vi "Initialize Motion.vi"(7 "Motion Control":T8={"SAS Geometry"=enum."Circular", "Angular Step"=1.0, "Vertical Step"=0.0, "Vertical Min"=0.0, "Vertical Max"=0.0, "Angular Start"=1.0, "Angular Stop"=20.0}, 8 "Error In":errorcluster, 11 "AirSAS Controls":T1={"Receive Duration"=0.0, "I/O"={"DAQmx Device"="Dev1", "AO Range"=0.0, "AI Range"=0.0, "DAQ Group Delay"=0.0, "Fs"=0.0}, "Hardware"={"Centerpos"=[], "TXpos"=[], "RX1pos"=[], "RX2pos"=[], "Angle"=0.0, "Height"=0.0}, "Waveform"={"LFM Parameters"={"Duration"=1.0, "Fstart (Hz)"=1000.0, "Fstop (Hz)"=10000.0, "Out. Amplitude (Vpk)"=1.0, "Window %"=10.0}, "Transmit Waveform"={"t0"=timestamp(0 s since 1904-01-01), "dt"=1.0, "Y"=[]}}, "LINX Resource"={"IO"=enum."Remote", "Interface"=enum."Serial", "LINX Device Config"={"Interface"=enum."Serial", "COM Port"="COM13", "TCP Configuration"={"IP Address"="", "Port"=0}, "Device Family"=1, "Device ID"=1, "Device Name"="myRIO-1900", "TCP Ref"=refnum, "Channels"={"DI"=[0, 1, 2, 3, 4, 5, 6, 7, 8, 9, 10, 11, 12, 13, 14, 15, 16, 17, 18, 19, 20, 21, 22, 23, 24, 25, 26, 27, 28, 29, 30, 31, 32, 33, 34, 35, 36, 37, 38, 39, 40, 41, 42, 43, 44, 45, 46], "DO"=[0, 1, 2, 3, 4, 5, 6, 7, 8, 9, 10, 11, 12, 13, 14, 15, 16, 17, 18, 19, 20, 21, 22, 23, 24, 25, 26, 27, 28, 29, 30, 31, 32, 33, 34, 35, 36, 37, 38, 39, 40, 41, 42, 43, 44, 45, 46], "AI"=[0, 1, 2, 3, 4, 5, 6, 7, 8, 9, 10, 11], "AO"=[], "PWM"=[3, 5, 6, 9, 10], "QE"=[], "UART"=[0, 1], "I2C 2"=[0], "SPI"=[0], "CAN"=[], "Servo"=[], "AI Ref (V)"=0.0, "AI Resolution (Bits)"=0, "AO Ref (V)"=0.0, "AO Resolution (Bits)"=0}}}, "Port"=3000.0} {"Waveform"."LFM Parameters"."Window %" format="%.2g"; "Waveform"."LFM Parameters"."Out. Amplitude (Vpk)" format="%0.2f"; "Waveform"."LFM Parameters"."Fstop (Hz)" format="%^.3e"; "Waveform"."LFM Parameters"."Fstart (Hz)" format="%^.3e"; "Waveform"."LFM Parameters"."Duration" format="%.3f"}) -> (0 "Error Out":errorcluster, 3 "output cluster":T1={"Receive Duration"=0.0, "I/O"={"DAQmx Device"="Dev1", "AO Range"=0.0, "AI Range"=0.0, "DAQ Group Delay"=0.0, "Fs"=0.0}, "Hardware"={"Centerpos"=[0.0, 0.0, 0.0], "TXpos"=[0.0, 0.0, 0.0], "RX1pos"=[0.0, 0.0, 0.0], "RX2pos"=[0.0, 0.0, 0.0], "Angle"=0.0, "Height"=0.0}, "Waveform"={"LFM Parameters"={"Duration"=1.0, "Fstart (Hz)"=1000.0, "Fstop (Hz)"=10000.0, "Out. Amplitude (Vpk)"=1.0, "Window %"=10.0}, "Transmit Waveform"={"t0"=timestamp(0 s since 1904-01-01), "dt"=1.0, "Y"=[]}}, "LINX Resource"={"IO"=enum."Remote", "Interface"=enum."Serial", "LINX Device Config"={"Interface"=enum."Serial", "COM Port"="COM13", "TCP Configuration"={"IP Address"="", "Port"=0}, "Device Family"=1, "Device ID"=1, "Device Name"="myRIO-1900", "TCP Ref"=refnum, "Channels"={"DI"=[0, 1, 2, 3, 4, 5, 6, 7, 8, 9, 10, 11, 12, 13, 14, 15, 16, 17, 18, 19, 20, 21, 22, 23, 24, 25, 26, 27, 28, 29, 30, 31, 32, 33, 34, 35, 36, 37, 38, 39, 40, 41, 42, 43, 44, 45, 46], "DO"=[0, 1, 2, 3, 4, 5, 6, 7, 8, 9, 10, 11, 12, 13, 14, 15, 16, 17, 18, 19, 20, 21, 22, 23, 24, 25, 26, 27, 28, 29, 30, 31, 32, 33, 34, 35, 36, 37, 38, 39, 40, 41, 42, 43, 44, 45, 46], "AI"=[0, 1, 2, 3, 4, 5, 6, 7, 8, 9, 10, 11], "AO"=[], "PWM"=[3, 5, 6, 9, 10], "QE"=[], "UART"=[0, 1], "I2C 2"=[0], "SPI"=[0], "CAN"=[], "Servo"=[], "AI Ref (V)"=0.0, "AI Resolution (Bits)"=0, "AO Ref (V)"=0.0, "AO Resolution (Bits)"=0}}}, "Port"=3000.0} {"Waveform"."LFM Parameters"."Window %" format="%.2g"; "Waveform"."LFM Parameters"."Out. Amplitude (Vpk)" format="%0.2f"; "Waveform"."LFM Parameters"."Fstop (Hz)" format="%^.3e"; "Waveform"."LFM Parameters"."Fstart (Hz)" format="%^.3e"; "Waveform"."LFM Parameters"."Duration" format="%.3f"})   [LabVIEW 2021]
uses:
  controls/Air SAS Controls.ctl
  <vilib>/MakerHub/LINX/Private/Type Defs/LINX Ref.ctl
  <vilib>/MakerHub/LINX/Private/Type Defs/Platform.ctl
  <vilib>/MakerHub/LINX/Private/Type Defs/Interface.ctl
  <vilib>/MakerHub/LINX/Private/Device/Type Defs/LINX Device Config.ctl
  <vilib>/MakerHub/LINX/Private/Device/Type Defs/TCP Config.ctl
  <vilib>/MakerHub/LINX/Private/Device/Type Defs/Channels.ctl
  <vilib>/MakerHub/LINX/LMH-LINX.lvlib
  <vilib>/MakerHub/LINX/Private/Device/Device.lvlib
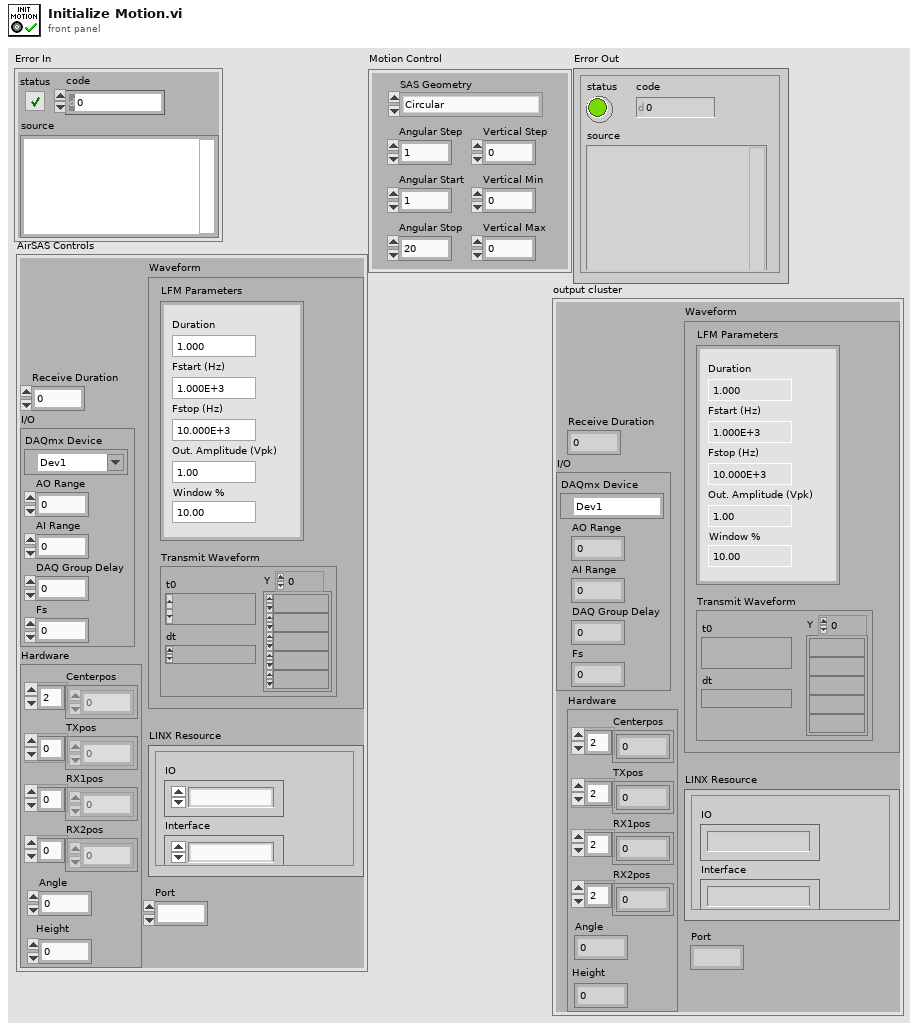
[diagram p1: front panel]
types:
  T1 = typedef "Air SAS Controls.ctl" = cluster{"Receive Duration":dbl, "I/O":cluster{"DAQmx Device":tag, "AO Range":dbl, "AI Range":dbl, "DAQ Group Delay":dbl, "Fs":dbl}, "Hardware":cluster{"Centerpos":dbl[], "TXpos":dbl[], "RX1pos":dbl[], "RX2pos":dbl[], "Angle":dbl, "Height":dbl}, "Waveform":cluster{"LFM Parameters":cluster{"Duration":dbl, "Fstart (Hz)":dbl, "Fstop (Hz)":dbl, "Out. Amplitude (Vpk)":dbl, "Window %":dbl}, "Transmit Waveform":waveform(dbl)}, "LINX Resource":T2, "Port":dbl}
  T2 = typedef "LMH-LINX.lvlib/LINX Ref.ctl" = cluster{"IO":T3, "Interface":T4, "LINX Device Config":T5}
  T3 = typedef "LMH-LINX.lvlib/Platform.ctl" = enum16{"Remote", "Local"}
  T4 = typedef "LMH-LINX.lvlib/Interface.ctl" = enum16{"Serial", "TCP"}
  T5 = typedef "LMH-LINX.lvlib/Device.lvlib/LINX Device Config.ctl" = cluster{"Interface":T4, "COM Port":refnum<visa-resource-name>, "TCP Configuration":T6, "Device Family":u8, "Device ID":u8, "Device Name":string, "TCP Ref":refnum<k5>, "Channels":T7}
  T6 = typedef "LMH-LINX.lvlib/Device.lvlib/TCP Config.ctl" = cluster{"IP Address":string, "Port":u16}
  T7 = typedef "LMH-LINX.lvlib/Channels.ctl" = cluster{"DI":u8[], "DO":u8[], "AI":u8[], "AO":u8[], "PWM":u8[], "QE":u8[], "UART":u8[], "I2C 2":u8[], "SPI":u8[], "CAN":u8[], "Servo":u8[], "AI Ref (V)":dbl, "AI Resolution (Bits)":u8, "AO Ref (V)":dbl, "AO Resolution (Bits)":u8}
  T8 = cluster{"SAS Geometry":enum16{"Circular", "Cylindrical", "Spiral"}, "Angular Step":dbl, "Vertical Step":dbl, "Vertical Min":dbl, "Vertical Max":dbl, "Angular Start":dbl, "Angular Stop":dbl}
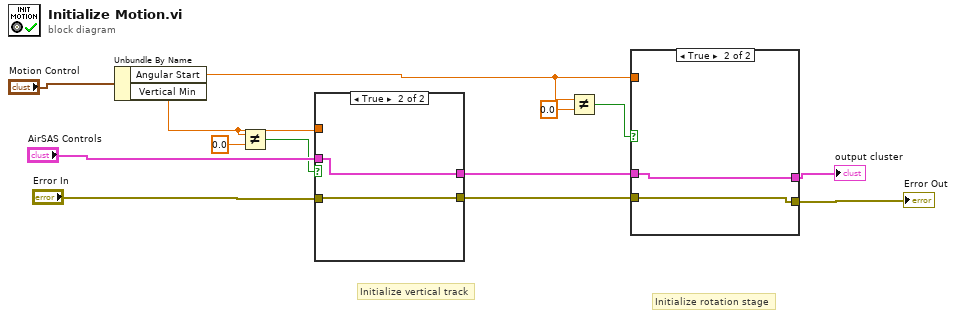
[diagram p0: block diagram]
diagram:
  # "Initialize rotation stage"
  # "Initialize vertical track"
  n1 = Unbundle By Name("Motion Control") -> ("Angular Start"=w3:dbl, "Vertical Min"=w6:dbl)
  n2 = Not Equal?(x=w6, y=0.0) -> (x != y?=w4:bool)
  n3 = case shown="True" w4 {
    tunnel: "Error In" -> [w14 w16]
    tunnel: "AirSAS Controls" -> [w15 w17]
    tunnel: [w15 w17] -> w11
    tunnel: [w14 w16] -> w10
    tunnel: w6 -> [_ _]
    frame False {
    }
    frame True {
    }
  }
  n4 = Not Equal?(x=w3, y=0.0) -> (x != y?=w1:bool)
  n5 = case shown="True" w1 {
    tunnel: w11 -> [w19 w21]
    tunnel: w10 -> [w18 w20]
    tunnel: w3 -> [_ _]
    tunnel: [w18 w20] -> w8
    tunnel: [w19 w21] -> w7
    frame False {
    }
    frame True {
    }
  }
  "Error Out" <- w8
  "output cluster" <- w7
